vi "Get Object Item by Name.vi"(7 "Item Name":string, 8 "error in (no error)":errorcluster, 10 "Object Offset":i32, 11 "JSON":string) -> (0 "error out":errorcluster, 1 "<JSON>":string caption="JSON substring", 2 "Item Offset (-1 if not found)":i32, 3 "Found":bool)   [LabVIEW 2013, in "JSONtext.lvlib"]
uses:
  JSONtext.lvlib
  support/JSONtext support.lvlib
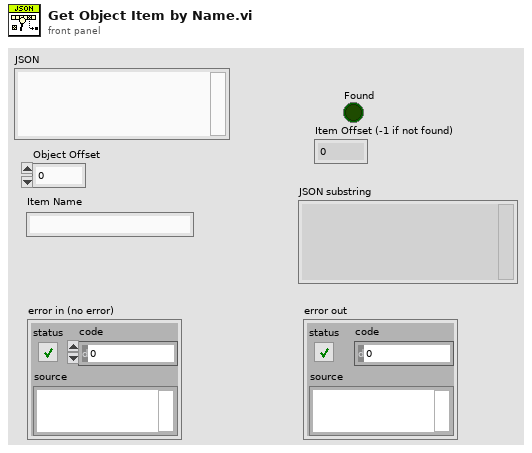
[diagram p1: front panel]
types:
  T1 = typedef "JSONtext.lvlib/JSON Value Search.ctl" = enum16{"Parser Error", "In Object", "In Array", "String", "Number", "Leading Whitespace", "Object end", "Array end", "Value end", "Undefined"}
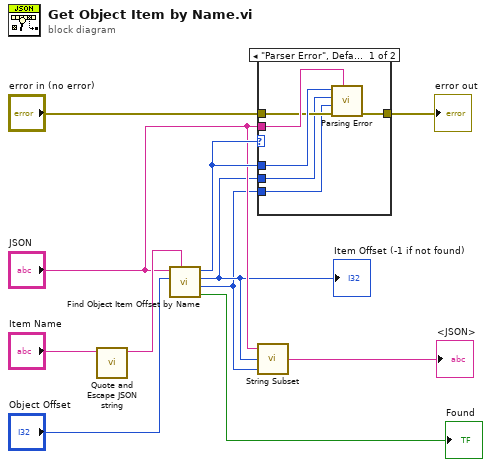
[diagram p0: block diagram]
diagram:
  n1 = call "Quote and Escape JSON string.vi"("Plain Text"="Item Name") -> ("<JSON>"=w6:string)  [unwired: 10 in]
  n2 = call "Find Object Item Offset by Name.vi"("Item Name <JSON>"=w6, "Object Offset"="Object Offset", "JSON"="JSON") -> ("Found"=→"Found":bool, "Offset past Item (or past last Item, if not found)"=w1:i32, "Item Offset (-1 if not found)"=w2:i32, "State"=w7:T1)  [unwired: 4 in, 1 out]
  "Item Offset (-1 if not found)" <- w2
  n3 = case shown="\"Parser Error\", Default" w7 {
    tunnel: w7 -> [w17 _]
    tunnel: "JSON" -> [w16 _]
    tunnel: "error in (no error)" -> [w15 w18]
    tunnel: [w14 w18] -> w4
    tunnel: w2 -> [w13 _]
    tunnel: w1 -> [w12 _]
    frame "Parser Error", Default {
      n4 = call "Parsing Error.vi"("JSON"=w16, "error in (no error)"=w15, "Offset past match"=w12, "Value start"=w13, "State"=w17) -> ("error out"=w14:errorcluster)  [unwired: 6 in]
    }
    frame "Value end" {
    }
  }
  "error out" <- w4
  n5 = call "String Subset.vi"("Offset past End"=w1, "Start offset"=w2, "JSON"="JSON") -> ("substring"=→"<JSON>":string)  [unwired: 2 in]
